vi "ZCAN_OpenDevice.vi"(8 "error in (no error)":errorcluster, 10 "device_index":u32, 11 "device_type":u32=41) -> (0 "error out":errorcluster, 1 "SerialNumber":string, 2 "DEVICE_INFO":string, 3 "DEVICE_HANDLE":u32)   [LabVIEW 2020, in "zlgcan.lvlib"]
uses:
  zlgcan.lvlib
  bin/zlgcan.dll
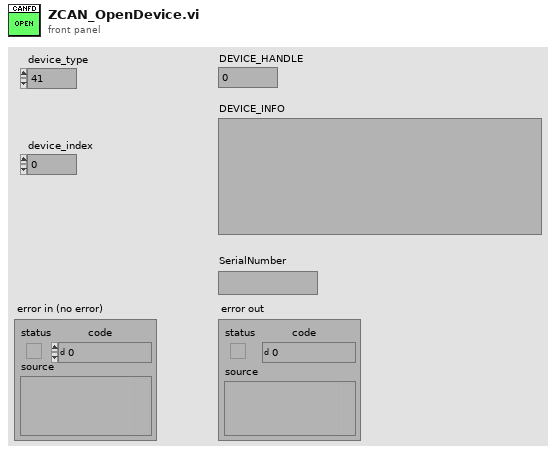
[diagram p1: front panel]
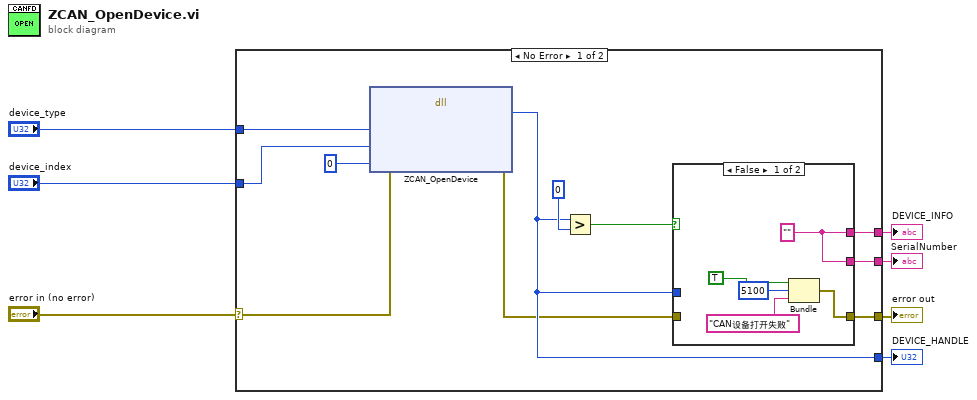
[diagram p0: block diagram]
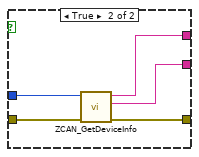
[diagram p2: hidden frame]
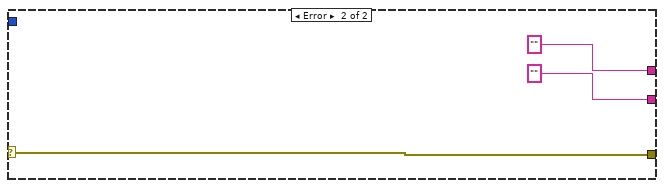
[diagram p3: hidden frame]
diagram:
  n1 = case shown="No Error" "error in (no error)" {
    selector: "error in (no error)" -> [w12 w31]
    tunnel: [w14 w31] -> w3
    tunnel: "device_type" -> [w18 _]
    tunnel: "device_index" -> [w17 _]
    tunnel: [w11 _] -> w5
    tunnel: [w10 "" ("DEVICE_INFO")] -> w2
    tunnel: [w9 "" ("SerialNumber")] -> w1
    frame No Error {
      n2 = dll-call lib="E:/Jabil tools/JabilTestLib/ZLG_CANFD/bin/zlgcan.dll" fn="ZCAN_OpenDevice"(error in=w12, "device_type"=w18, "device_index"=w17, "reserved"=u32 0) -> (error out=w8:errorcluster, "DEVICE_HANDLE"=w11:u32)  [unwired: 5 in, 1 out]
      n3 = Greater?(x=w11, y=u32 0) -> (0:w15:bool)
      n4 = case shown="False" w15 {
        tunnel: [w22 w27] -> w14
        tunnel: w11 -> [_ w28]
        tunnel: [w19 w26] -> w10
        tunnel: [w19 w25] -> w9
        tunnel: w8 -> [_ w24]
        frame False {
          w19 = "" ("DEVICE_INFO")
          n5 = Bundle("status"=TRUE, "code"=5100, "消息"="CAN设备打开失败") -> (w22:cluster{"status":bool, "code":i32, "消息":string})  [unwired: 1 in]
        }
        frame True {
          n6 = call "ZCAN_GetDeviceInfo.vi"("DEVICE_HANDLE"=w28, "error in (no error)"=w24) -> ("DEVICE_INFO"=w26:string, "SerialNumber"=w25:string, "error out"=w27:errorcluster)  [unwired: 4 in]
        }
      }
    }
    frame Error {
    }
  }
  "DEVICE_HANDLE" <- w5
  "error out" <- w3
  "DEVICE_INFO" <- w2
  "SerialNumber" <- w1
